vi "read_data.vi"(8 "error in (no error)":errorcluster, 11 "Mixture in":refnum<class "Mixture.lvclass">) -> (0 "error out":errorcluster, 2 "data":T1={"n_samples"=1.0}, 3 "Mixture out":refnum<class "Mixture.lvclass">)   [LabVIEW 2020, in "Mixture.lvclass"]
uses:
  Mixture.lvclass
  Controls/mixture_data.ctl
  Mixture.lvclass/Mixture.ctl
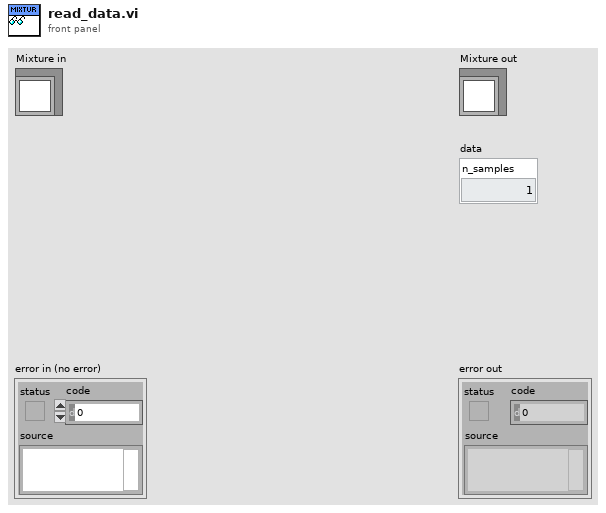
[diagram p1: front panel]
types:
  T1 = typedef "mixture_data.ctl" = cluster{"n_samples":dbl}
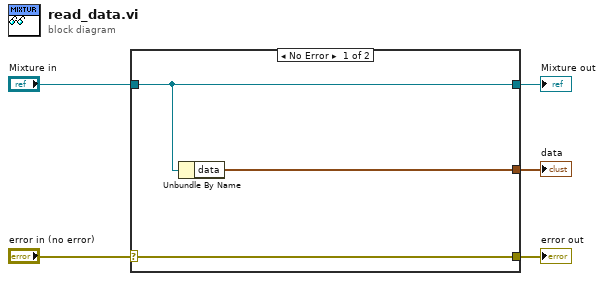
[diagram p0: block diagram]
diagram:
  n1 = case shown="No Error" "error in (no error)" {
    selector: "error in (no error)" -> [w8 w9]
    tunnel: [w8 w9] -> w4
    tunnel: [w7 w10] -> w2
    tunnel: "Mixture in" -> [w7 w10]
    tunnel: [w6 _] -> w1
    frame No Error {
      n2 = Unbundle By Name(w7) -> ("data"=w6:T1)
    }
    frame Error {
    }
  }
  "error out" <- w4
  "Mixture out" <- w2
  "data" <- w1
